vi "Read FP Tags.vi"(8 "error in (no error)":errorcluster, 11 "Context in":T1) -> (0 "error out":errorcluster, 3 "Context out":T1)   [LabVIEW 2020, in "DocTool.lvlib"]
uses:
  DocTool.lvlib
  TDefs/Context.ctl
  Events.ctl
  UserEvent.ctl
  TDefs/State.ctl
  TDefs/States.ctl
  TDefs/Single File Properties.ctl
  TDefs/FP Items Properties.ctl
  TDefs/FP Item Properties.ctl
  TDefs/CopyTag.ctl
  StateMachine.lvlib
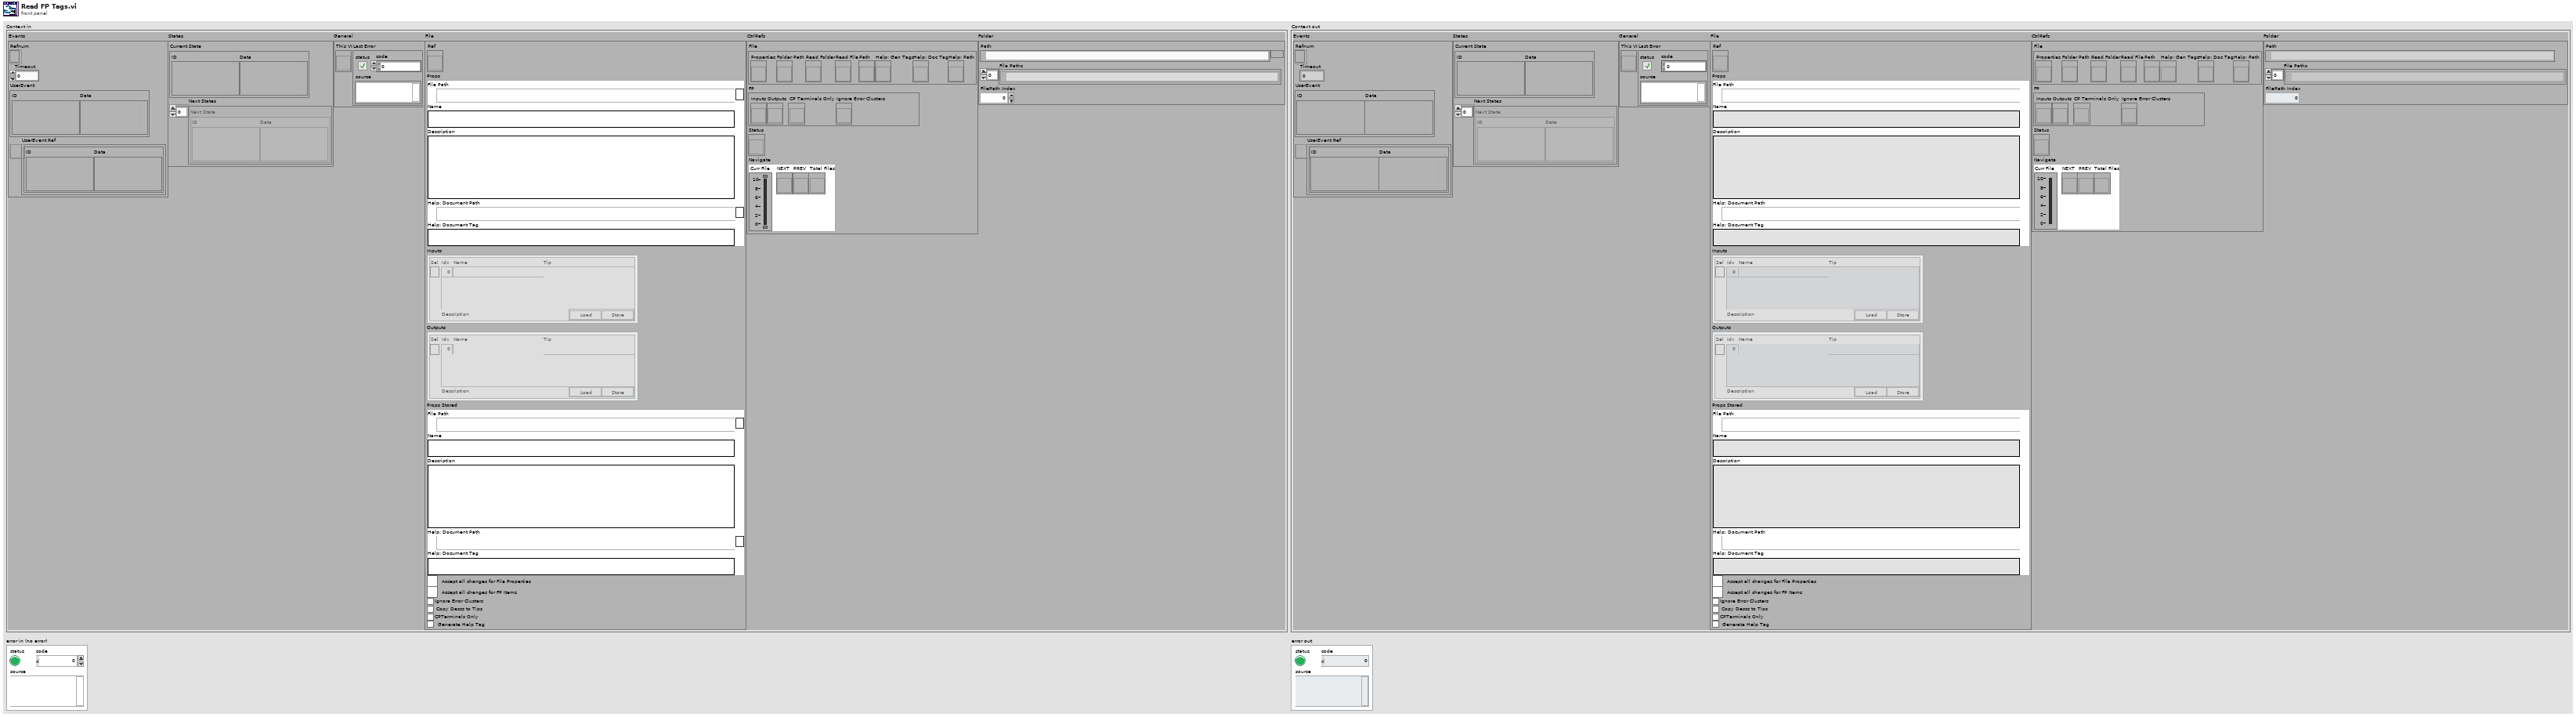
[diagram p1: front panel]
types:
  T1 = typedef "DocTool.lvlib/Context.ctl" = cluster{"Events":T2, "States":cluster{"Current State":T4, "Next States":T5}, "General":cluster{"This VI":refnum<vi>, "Last Error":errorcluster}, "File":cluster{"Ref":refnum<vi>, "Props":T6, "Inputs":T7, "Outputs":T7, "Props Stored":T6, "Write":bool, "Write FP":bool, "Ignore Error Clusters":bool, "Copy Descs to Tips":bool, "CPTerminals Only":bool, "Generate Help Tag":bool}, "CtrlRefs":cluster{"File":cluster{"Properties":refnum<vi>, "Folder Path":refnum<vi>, "Read Folder":refnum<vi>, "Read File":refnum<vi>, "Path":refnum<vi>, "Help: Gen Tags":refnum<vi>, "Help: Doc Tag":refnum<vi>, "Help: Path":refnum<vi>}, "FP":cluster{"Inputs":refnum<vi>, "Outputs":refnum<vi>, "CP Terminals Only":refnum<vi>, "Ignore Error Clusters":refnum<vi>}, "Status":refnum<vi>, "Navigate":cluster{"Curr File":refnum<vi>, "NEXT":refnum<vi>, "PREV":refnum<vi>, "Total Files":refnum<vi>}}, "Folder":cluster{"Path":path, "File Paths":path[], "FilePath Index":i32}}
  T2 = typedef "StateMachine.lvlib/Events.ctl" = cluster{"Refnum":refnum<event-registration>, "Timeout":i32, "UserEvent":T3, "UserEvent Ref":refnum<user-event>}
  T3 = typedef "StateMachine.lvlib/UserEvent.ctl" = cluster{"ID":variant, "Data":variant}
  T4 = typedef "StateMachine.lvlib/State.ctl" = cluster{"ID":variant, "Data":variant}
  T5 = typedef "StateMachine.lvlib/States.ctl" = T4[]
  T6 = typedef "DocTool.lvlib/Single File Properties.ctl" = cluster{"File Path":path, "Name":string, "Description":string, "Help: Document Path":path, "Help: Document Tag":string}
  T7 = typedef "DocTool.lvlib/FP Items Properties.ctl" = T8[]
  T8 = typedef "DocTool.lvlib/FP Item Properties.ctl" = cluster{"Sel":bool, "Idx":i32, "Name":string, "Description":string, "Tip":string, "Load Store":T9}
  T9 = typedef "DocTool.lvlib/CopyTag.ctl" = cluster{"Load":bool, "Store":bool}
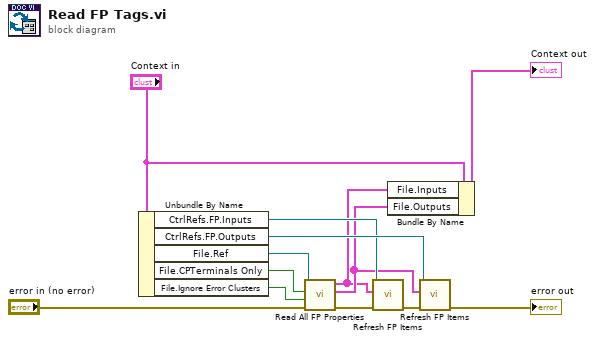
[diagram p0: block diagram]
diagram:
  n1 = Unbundle By Name("Context in") -> ("CtrlRefs.FP.Inputs"=w7:refnum<vi>, "CtrlRefs.FP.Outputs"=w8:refnum<vi>, "File.Ref"=w6:refnum<vi>, "File.CPTerminals Only"=w5:bool, "File.Ignore Error Clusters"=w4:bool)
  n2 = call "Read All FP Properties.vi"("error in (no error)"="error in (no error)", "No Error clusters"=w4, "Is On Connector Pane"=w5, "VI in"=w6) -> ("error out"=w11:errorcluster, "Outputs"=w3:T7, "Inputs"=w2:T7)  [unwired: 5 in]
  n3 = call "Refresh FP Items.vi"("error in (no error)"=w11, "FP Item Props in"=w2, "Array in"=w7) -> ("error out"=w1:errorcluster)  [unwired: 8 in]
  n4 = Bundle By Name(cluster="Context in", "File.Inputs"=w2, "File.Outputs"=w3) -> (→"Context out":T1)
  n5 = call "Refresh FP Items.vi"("error in (no error)"=w1, "FP Item Props in"=w3, "Array in"=w8) -> ("error out"=→"error out":errorcluster)  [unwired: 8 in]
